vi "Set Osc Channel Range.vi"(9 "maxmv":i32, 10 "minmv":i32, 11 "channel":i32) -> (3 "function return":i32)   [LabVIEW 2021, in "vmmso.lvlib"]
doc: "DLL_API int WINAPI SetOscChannelRange(int channel, int minmv, int maxmv);"
uses:
  vmmso.lvlib
  vmmso.dll
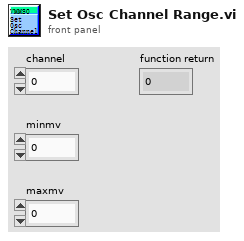
[diagram p1: front panel]
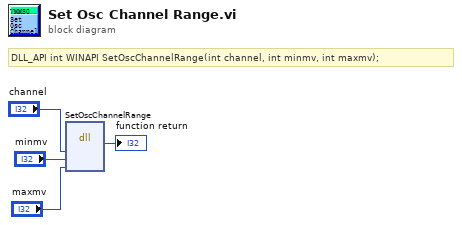
[diagram p0: block diagram]
diagram:
  # "DLL_API int WINAPI SetOscChannelRange(int channel, int minmv, int maxmv);"
  n1 = dll-call lib="D:/labviewdemo/LabviewDemo 21/vmmso/vmmso.*" fn="SetOscChannelRange"("channel"="channel", "minmv"="minmv", "maxmv"="maxmv") -> (→"function return":i32)  [unwired: 6 in, 2 out]
